vi "getGraph.vi"(0 "Cam_Calib_file":path, 1 "Spec_Calib_file":path, 3 "ROI":bool, 4 "map":path, 5 "y0":i32, 6 "FW":bool, 7 "image in":path, 9 "cam (0,1,2,3)":i32, 10 "Lens":string(combo)="f8x06", 11 "Image Name":string, 12 "B [T]":dbl=1.0) -> (13 "output cluster":cluster{"dp [MeV/C]":dbl[], dbl[]}(graph), 14 "Y":dbl[][](array[numeric]), 15 "X":dbl[][](array[numeric]), 17 "Momentum [MeV/C]":dbl[](graph), 18 "z":dbl[][](array[numeric]), 19 "pixel angel (y)":dbl[](graph)=[0.28800769934064135, 0.2882095085032147, 0.2884115340157437, 0.28861377619454537, 0.2888162353565284, 0.2890189118191943, 0.2892218059006397, 0.289423234715329, 0.2896096026494926, 0.2897858413876203, 0.28996224180170876, 0.29013880409125165, 0.2903155284560538, 0.2904924150962318, 0.29066946421221485, 0.2908466760047451, 0.2910240506748785, 0.2912200888475889, 0.29142082546369963, 0.29162177442700027, 0.2918229360446737, 0.29202431062447265, 0.2922258984747208, 0.29242769990431444, 0.2926297152227232, 0.29283191570579953, 0.2930334377606523, 0.2932351725330019, 0.2934371203297612, 0.2936387877464904, 0.2938402641743795, 0.2940419529321517, 0.2942438543260385, 0.29444596866283795, 0.2946480589358109, 0.29484968035757747, 0.29505151355782316, 0.2952535588408159, 0.2954558165113846, 0.29565828687491924, 0.2958609702373737, 0.2960638669052662, 0.2962669771856805, 0.2964698040291343, 0.2966723158133113, 0.2968750398090262, 0.2970779763202955, 0.2972811256516943, 0.29748448810835737, 0.29768806399598025, 0.29789287923215024, 0.29809853177062107, 0.2982861778747611, 0.2984666288230578, 0.2986472437516359, 0.29882802286022364, 0.2990089663488561, 0.2991900744178752, 0.29937134726793113, 0.2995527850999821, 0.29973438811529546, 0.2999384554163026, 0.3001441852119658, 0.30035013071239275, 0.30055629222582286, 0.300762670061059, 0.3009692645274684, 0.3011760759349845, 0.3013831045941078, 0.30159015680064977, 0.30179572710684616, 0.3019980055244977, 0.3022004922691996, 0.30240318763470797, 0.30260609191531024, 0.3028092054058265, 0.30301252840161114, 0.30321606119855377, 0.3034193370385415, 0.303622099252708, 0.3038250695143296, 0.30402824811549045, 0.30423163534880104, 0.30443523150739876, 0.3046390368849498, 0.3048430517756495, 0.30504727647422436, 0.305250926214299, 0.30545430210508306, 0.30565724830341984, 0.3058593076106099, 0.3060615723804524, 0.3062640428992535, 0.3064667194538319, 0.30666960233151963, 0.3068726918201636, 0.3070747819785802, 0.3072768576621269, 0.30747913769575613, 0.30768162236242985, 0.30788431194561355, 0.30808720672927653, 0.3082903069978933, 0.3084936130364445, 0.3086970146579123, 0.30889922498337297, 0.3091016386512774, 0.30930519276357565, 0.30950964116951185, 0.30971429656540866, 0.30991915923741287, 0.31012422947217805, 0.31032950755686545, 0.31052667203082357, 0.3107046103456832, 0.31088270164873605, 0.31106094611610596, 0.31123934392417213, 0.31141789524956964, 0.3115966002691897, 0.31177545916018046, 0.3119544720999468, 0.31214640622298384, 0.31234998693136795, 0.31255336482074314, 0.31275519333119467, 0.31295722155025546, 0.31315944974786275, 0.3133618781944213, 0.31356450716080464, 0.3137673369183555, 0.3139684633147784, 0.3141691648118955, 0.31437006254733935, 0.31457115678279784, 0.31477244778040603, 0.3149739358027459, 0.3151756211128486, 0.31537750397419384, 0.3155795846507125, 0.3157784918983376, 0.3159787797187646, 0.31617965487765226, 0.31638072445801957, 0.31658198871544435, 0.31678344790593305, 0.3169851022859213, 0.3171869521122753, 0.317387977202208, 0.3175852989941981, 0.31778280689627375, 0.3179805011460661, 0.3181783819815921, 0.31837644964125583, 0.31857470436384855, 0.3187731463885496, 0.31897177595492787, 0.319164425005991, 0.3193518219719201, 0.3195393858305189, 0.3197271167829648, 0.319915015030744, 0.32010308077565147, 0.32029131421979173, 0.32047971556557964, 0.3206682850157408, 0.3208688467868947, 0.3210756600957864, 0.3212826784341325, 0.3214899020805093, 0.3216973313139795, 0.3219049664140931, 0.3221128076608881, 0.32232085533489246, 0.322529109717124, 0.3227113886977328, 0.3228905273030448, 0.3230698154730057, 0.3232492533752553, 0.3234288411776704, 0.3236085790483658, 0.3237884671556941, 0.3239685056682464, 0.3241511143038239, 0.3243524891978669, 0.3245540552936161, 0.3247552106478079, 0.3249552231079993, 0.32515542436888734, 0.32535581467399116, 0.32555639426723304, 0.32575716339293825, 0.32596597642227865, 0.3261901232146414, 0.3264145104321994, 0.3266391384324378, 0.32686400757353024, 0.3270891182143402, 0.327314470714423, 0.32754006543402703, 0.32776590273409556, 0.32799189932134853, 0.3282180755480182, 0.32844449509892426, 0.32867115833698873, 0.3288980656258346, 0.3291252173297875, 0.32935261381387765, 0.32958025544384106, 0.32980814258612173, 0.330028974231201, 0.33024815924312484, 0.33046756988987364, 0.3306872937363768, 0.3309074671757531, 0.33112786774508135, 0.33134849576745934, 0.3315693515665783, 0.331790255775179, 0.3320036146728935, 0.3322171849209621, 0.33243096680671685, 0.33264496061799237, 0.3328591666431264, 0.33307358517096125, 0.333288216490845, 0.3335030608926323, 0.3337238815649635, 0.33396228506727366, 0.3342009553991622, 0.3344398929760186, 0.3346790982140716, 0.3349185715303916, 0.335158313342892, 0.33539832407033227, 0.3356386041323192, 0.33586336923097243, 0.3360709979838858, 0.33627882311063856, 0.3364836936146091, 0.3366885950037914, 0.33689368820826937, 0.3370989734740675, 0.33730445104761525, 0.33751012117574847, 0.3377137462769637, 0.3379166145664905, 0.33811966975822294, 0.3383229120876115, 0.3385263417904872, 0.3387299591030621, 0.33893376426193, 0.3391377575040679, 0.3393419390668357, 0.33957117083159105, 0.3398025156289204, 0.3400341070851385, 0.3402659455657455, 0.3404980314369444, 0.3407303650656422, 0.34096294681945183, 0.3411957770666942, 0.34142339852169173, 0.3416239795756783, 0.341824740848181, 0.3420256825600719, 0.34222680493256974, 0.34242810818724057, 0.34262959254599806, 0.3428312582311045, 0.3430331054651715, 0.34323429066279754, 0.3434343003072502, 0.3436344879226952, 0.3438348537248517, 0.3440353979297727, 0.3442361207538469, 0.3444370224137983, 0.3446381031266871, 0.34483936310991076, 0.3450578626541485, 0.3452874643561488, 0.3455173043193103, 0.34574732020818016, 0.3459723897434692, 0.3461976898022912, 0.34642322071410303, 0.346648982808974, 0.34687497641758697, 0.34707394456279084, 0.34726779758963844, 0.3474618167179976, 0.3476560021425361, 0.34785035405821507, 0.34804487266028833, 0.34823955814430335, 0.3484344107061026, 0.3486312649180983, 0.34885495465101213, 0.3490788695629513, 0.3493030099695635, 0.34952737618707086, 0.3497519685322719, 0.34997731548961586, 0.35020527925995326, 0.35043347490544124, 0.35065231866296387, 0.3508480345697342, 0.3510439168590296, 0.3512399657230985, 0.3514361813544731, 0.3516325639459694, 0.3518291136906883, 0.3520258307820155, 0.3522227154136226, 0.35241870033027983, 0.35261385771009734, 0.3528091794518836, 0.35300466574353223, 0.3532003167732107, 0.3533961327293609, 0.35359211380069955, 0.35378793248579343, 0.3539823127088366, 0.35419856946847766, 0.3544224703728747, 0.3546465920460918, 0.3548709347899404, 0.3550954989067666, 0.35532028469945204, 0.355545292471415, 0.3557705225266119, 0.35599597516953835, 0.3562195465688293, 0.35644327578022983, 0.3566672238740321, 0.35689139114683444, 0.35711577789575555, 0.35734038441843524, 0.357565211013036, 0.3577868369248013, 0.3579969740834651, 0.3581801509931798, 0.3583634719989251, 0.35854693725604614, 0.3587305469201026, 0.35891430114686995, 0.35909820009233984, 0.35928224391272, 0.35946643276443463, 0.35966343275620455, 0.3598777096374909, 0.36009218772835716, 0.3603068672927925, 0.3605217485952368, 0.3607368319005817, 0.36095458016808163, 0.36117878865288006, 0.3614032134202907, 0.36160546206413874, 0.36179594817013894, 0.3619865861077824, 0.36217737604056577, 0.36236831813220927, 0.362559412546657, 0.36275065944807766, 0.3629420590008647, 0.36313361136963646, 0.363351808428183, 0.3635738459612016, 0.36379609356232473, 0.3640185515055202, 0.36423767597445017, 0.364450336432046, 0.36466319251442797, 0.36487624447297334, 0.36508925281984417, 0.36530043816401897, 0.365511815657225, 0.36572338554338923, 0.36593514806684124, 0.3661471034723142, 0.3663592520049456, 0.3665715939102782, 0.3667841294342608, 0.3669960968480711, 0.367206729858304, 0.3674198832826266, 0.3676334264586519, 0.36784716366746734, 0.3680610951539646, 0.3682752211634362, 0.3684895419415763, 0.36870405773448195, 0.36889898923916287, 0.36907852436519195, 0.3692581922210982, 0.3694379929399495, 0.36961792665498383, 0.36979799349960923, 0.36997791071534186, 0.37015298423759135, 0.37032818465487666, 0.370527824153792, 0.370734224899929, 0.37094080653068184, 0.37114756926726766, 0.3713545133312559, 0.3715616389445682, 0.3717689463294794, 0.3719764357086188, 0.3721840747166905, 0.3723895491590272, 0.3725955361453253, 0.37280376147382954, 0.3730121687603038, 0.37322075822564516, 0.3734295300910985, 0.3736384845782571, 0.37384762190906357, 0.37405635571757884, 0.3742634182839463, 0.37447065975982285, 0.37467808035967864, 0.37488568029831626, 0.3750934597908729, 0.3753031816848105, 0.37551380655424726, 0.37572461515960376, 0.3759344528378446, 0.37614315553648375, 0.37635203799113537, 0.3765611004155991, 0.3767703430240029, 0.3769797660308043, 0.37718936965079053, 0.37739915409907876, 0.3776091195911178, 0.3778123048177794, 0.3780130727617814, 0.3782140080126384, 0.37841511076446727, 0.3786163812116777, 0.3788178195489723, 0.3790194259713473, 0.37922120067409315, 0.37942314385279496, 0.37959132786416794, 0.3797567204840217, 0.37992360723587615, 0.3800914896866685, 0.38025948438880225, 0.3804275914436931, 0.3805958109528732, 0.380764143017991, 0.38093731804963116, 0.3811378564602311, 0.38133855908668424, 0.3815394261150738, 0.3817404577317556, 0.38194370958430596, 0.38214741221894494, 0.3823512831791136, 0.3825553226566906, 0.3827585341269448, 0.38296024944966484, 0.3831621291366564, 0.3833641733723683, 0.3835663823415161, 0.38376875622908285, 0.3839664488014421, 0.38415997372343197, 0.38435365206763583, 0.3845668564899877, 0.38479308272283114, 0.38501952376050674, 0.3852461798925063, 0.3854730514088339, 0.3857001386000069, 0.3859274417570573, 0.3861568553104828, 0.3863866526183244, 0.3865851388515057, 0.3867772598985196, 0.3869695298488373, 0.3871619488624852, 0.3873545170997119, 0.3875472347209896, 0.38774010188701397, 0.38793081685388153, 0.38812024927651523, 0.3883072180685801, 0.3884943280128661, 0.3886815792576781, 0.38886897195152265, 0.38905650624310933, 0.3892441822813508, 0.38943200021536284, 0.3896199601944651, 0.3898072824309816, 0.3899927621065785, 0.39017837977852254, 0.39036413558945854, 0.39055002968222213, 0.39073606219984064, 0.39092223328553327, 0.39110717852291554, 0.39129003029545684, 0.3914716422770283, 0.39165206132783087, 0.39183261109100753, 0.3920132916986519])   [LabVIEW 2011]
uses:
  <vilib>/vision/NI_Vision_Development_Module.lvlib
panel:
  out "Image Pixels (I16)":i16[][](graph)
  out "start":dbl
  in  "Cluster":cluster{"0":i32, "1":i32, "2":i32, "3":i32}
  out "x/y":dbl[][](graph)
  out "filenames":string[](array[string])
  out "Image Dst Out":T1(plugin-control)
  out "Y Resolution":i32
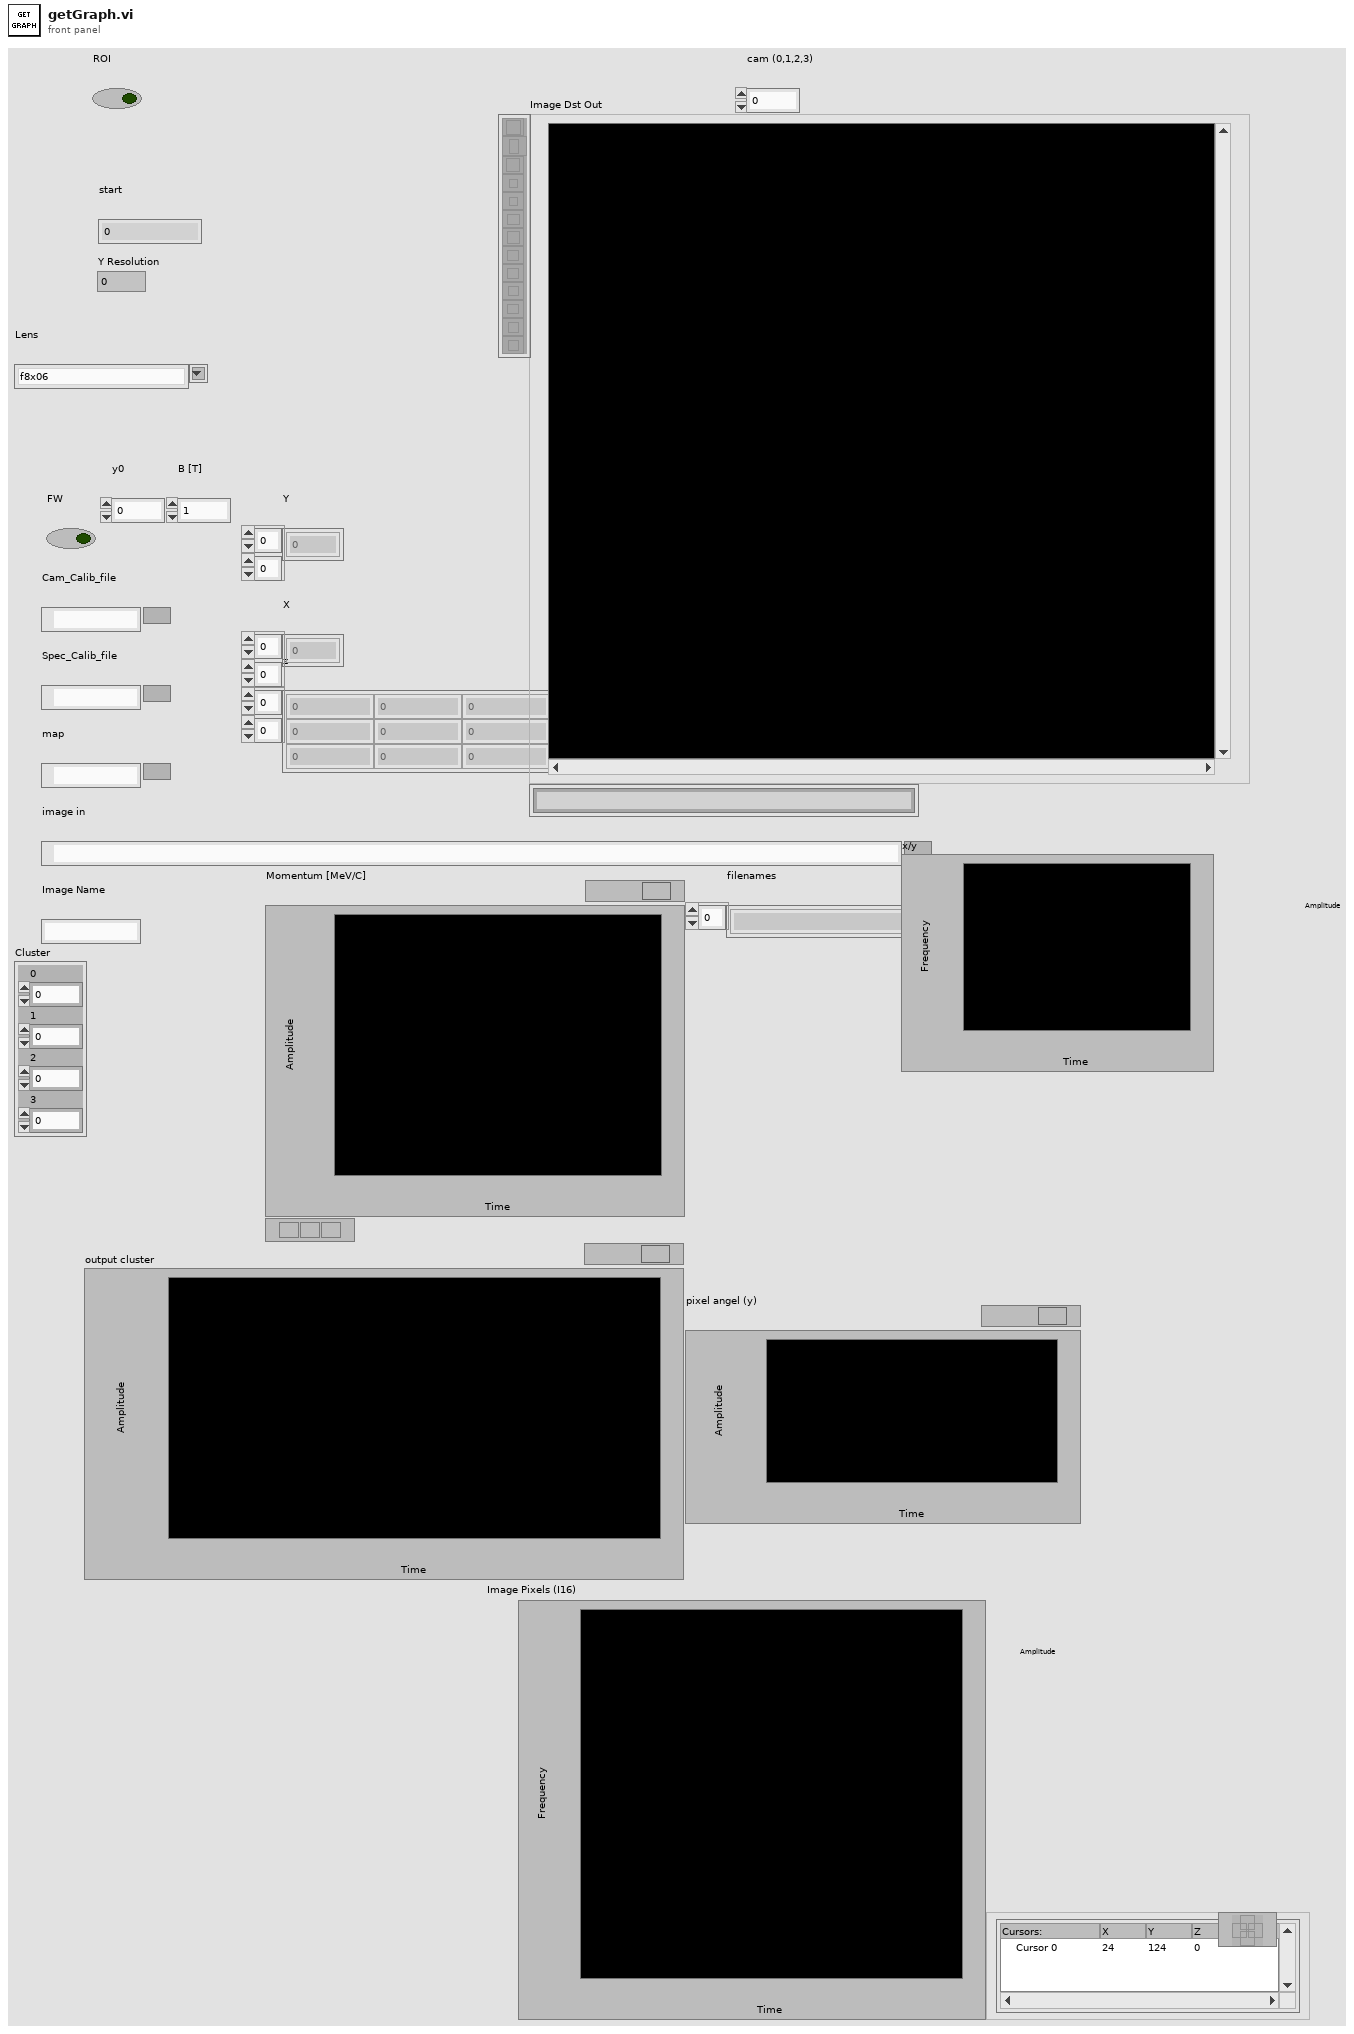
[diagram p1: front panel]
types:
  T1 = typedef "IMAQ Image.ctl" = refnum<image>
  T2 = cluster{"X Size":i32, "Y Size":i32, "Order #":i32}
  T3 = cluster{"npix-X":i32, "npix-Y":i32, "Left [pix]":dbl, "Top [pix]":dbl}
  T4 = cluster{"Screen Orientation":string, "Screen angle":string, "Lens":string, "Calibration (mm/pix)":dbl}
  T5 = typedef "Image Type" = u32
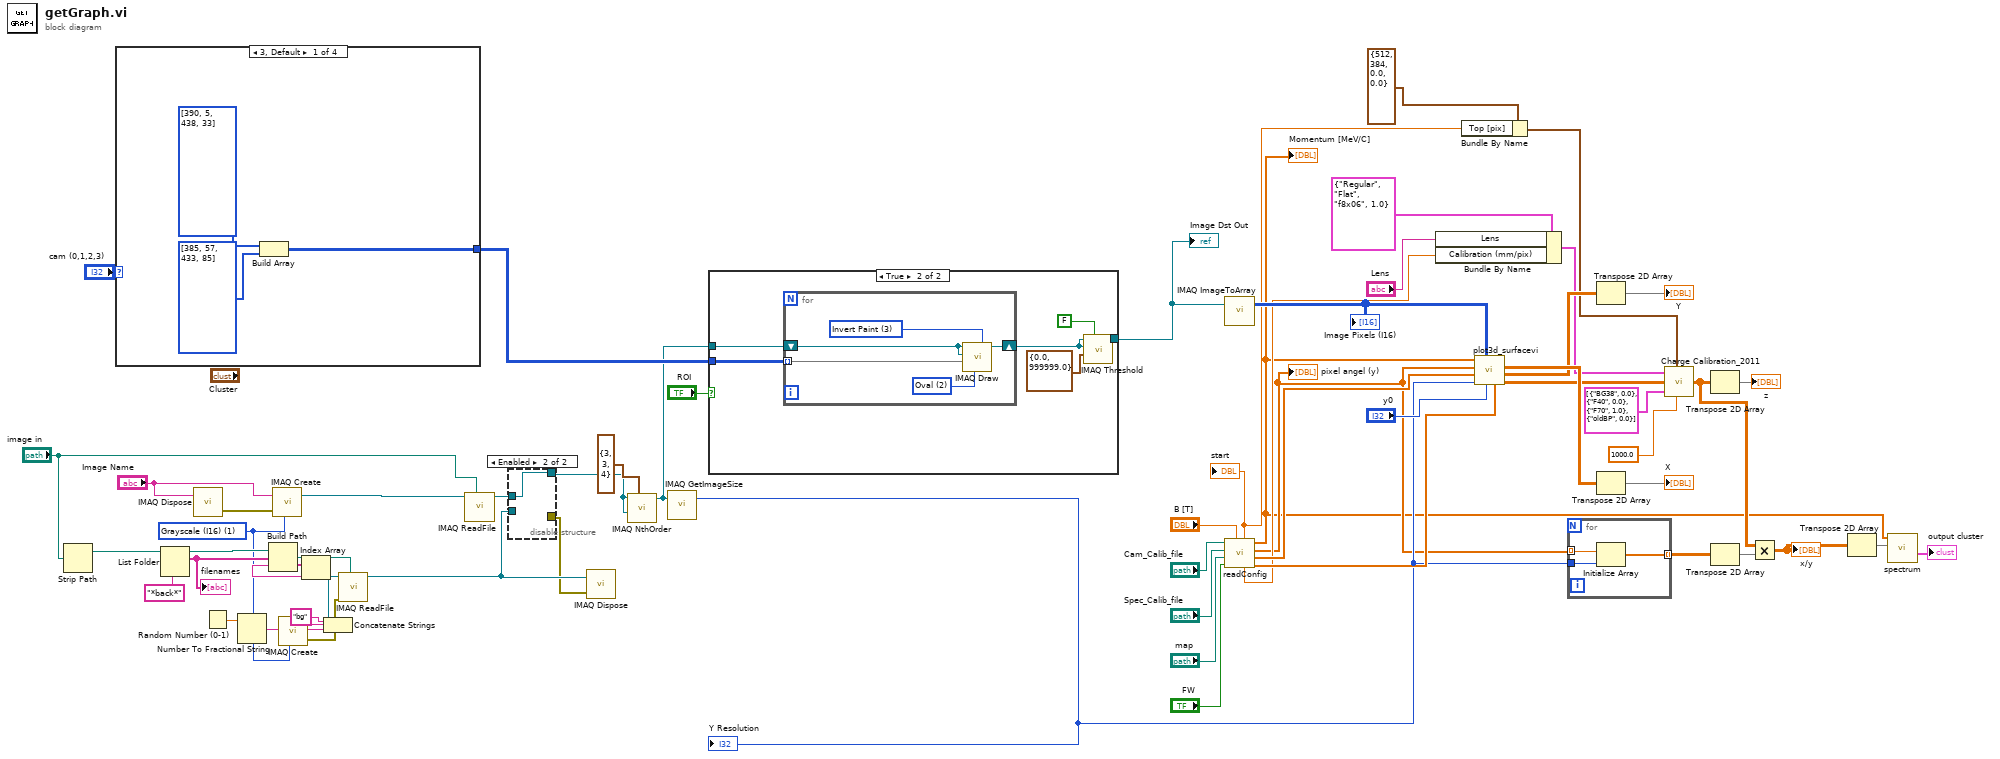
[diagram p0: block diagram]
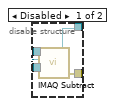
[diagram p2: hidden frame]
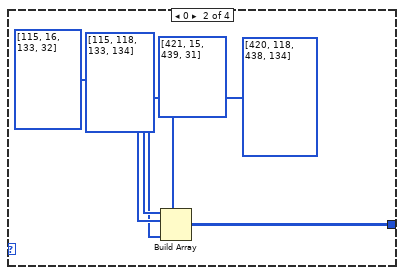
[diagram p3: hidden frame]
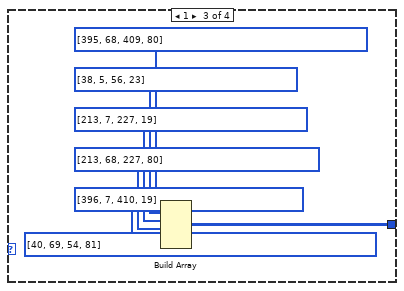
[diagram p4: hidden frame]
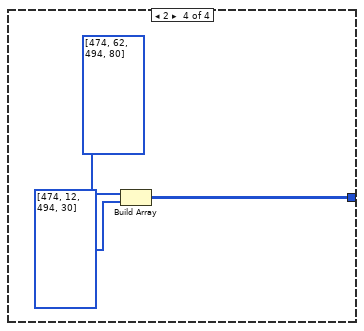
[diagram p5: hidden frame]
diagram:
  w22 = T5 1 items=["Grayscale (U8)", "Grayscale (I16)", "Grayscale (SGL)", "Complex (CSG)", "RGB (U32)", "HSL (U32)", "RGB (U64)", "Grayscale (U16)"] ("Image Type")
  n1 = Strip Path(path="image in") -> (stripped path=w31:path)  [unwired: 1 out]
  n2 = case shown="3, Default" "cam (0,1,2,3)" {
    tunnel: [w61 w66 w73 w76] -> w13
    frame 3, Default {
      n3 = Build Array(i32[] [390, 5, 438, 33] ("Points"), i32[] [385, 57, 433, 85] ("Points")) -> (w61:i32[][])
    }
    frame 0 {
      n4 = Build Array(i32[] [115, 16, 133, 32] ("Global Rectangle"), i32[] [115, 118, 133, 134] ("Global Rectangle"), i32[] [421, 15, 439, 31] ("Global Rectangle"), i32[] [420, 118, 438, 134] ("Global Rectangle")) -> (w66:i32[][])
    }
    frame 1 {
      n5 = Build Array(i32[] [395, 68, 409, 80] ("Global Rectangle"), i32[] [38, 5, 56, 23] ("Global Rectangle"), i32[] [213, 7, 227, 19] ("Global Rectangle"), i32[] [213, 68, 227, 80] ("Global Rectangle"), i32[] [396, 7, 410, 19] ("Global Rectangle"), i32[] [40, 69, 54, 81] ("Global Rectangle")) -> (w73:i32[][])
    }
    frame 2 {
      n6 = Build Array(i32[] [474, 62, 494, 80] ("Points"), i32[] [474, 12, 494, 30] ("Points")) -> (w76:i32[][])
    }
  }
  n7 = List Folder(path=w31, pattern="*back*") -> (path out=w28:path, filenames=w29:string[])  [unwired: 2 in, 2 out]
  "filenames" <- w29
  n8 = call "IMAQ Dispose"("Image"="Image Name") -> ("error out"=w54:errorcluster)  [unwired: 5 in]
  n9 = Random Number (0-1)() -> (number: 0 to 1=w26:dbl)
  n10 = Number To Fractional String(number=w26) -> (F-format string=w24:string)  [unwired: 3 in]
  n11 = call "IMAQ Create"("Image Name"="Image Name", "Image Type"=w22, "error in (no error)"=w54) -> ("New Image"=w52:T1)  [unwired: 2 in, 1 out]
  n12 = Index Array(array=w29) -> (element=w27:string)  [unwired: 1 in]
  n13 = Build Path(base path=w28, name or relative path=w27) -> (appended path=w20:path)
  n14 = Concatenate Strings("bg" ("Image Name"), w24) -> (w23:string)
  n15 = call "IMAQ Create"("Image Name"=w23, "Image Type"=w22) -> ("New Image"=w21:T1, "error out"=w17:errorcluster)  [unwired: 3 in]
  n16 = call "IMAQ ReadFile"("File Path"=w20, "error in (no error)"=w17, "Image"=w21) -> ("Image Out"=w16:T1)  [unwired: 4 in, 4 out]
  n17 = call "IMAQ ReadFile"("File Path"="image in", "Image"=w52) -> ("Image Out"=w19:T1)  [unwired: 5 in, 4 out]
  n18 = disable-structure shown="Enabled" {
    disable-tunnel: w19 -> [w82 w83]
    disable-tunnel: [w81 w83] -> w18
    disable-tunnel: w16 -> [w80 _]
    disable-tunnel: [w79 _] -> w15
    frame Disabled {
      n19 = call "IMAQ Subtract"("Image Src A"=w82, "Image Dst"=w82, "Image Src B"=w80) -> ("Image Dst Out"=w81:T1, "error out"=w79:errorcluster)  [unwired: 4 in]
    }
    frame Enabled {
    }
  }
  n20 = call "IMAQ Dispose"("Image"=w16, "error in (no error)"=w15) -> ()  [unwired: 4 in, 1 out]
  n21 = call "IMAQ NthOrder"("Image Src"=w18, "Size & Order #"=T2 {"X Size"=3, "Y Size"=3, "Order #"=4}, "Image Dst"=w18) -> ("Image Dst Out"=w1:T1)  [unwired: 4 in, 1 out]
  n22 = call "IMAQ GetImageSize"("Image"=w1) -> ("Y Resolution"=w12:i32)  [unwired: 3 in, 2 out]
  "Y Resolution" <- w12
  n23 = case shown="True" "ROI" {
    tunnel: w1 -> [w84 w88]
    tunnel: [w84 w87] -> w2
    tunnel: w13 -> [_ w85]
    frame False {
    }
    frame True {
      n24 = for {
        shift-right: [w94] -> w86
        shift-left: w88 -> [w95]
        tunnel: w85 -> [w91] mode=indexing
        w93 = u16 2 items=["Line", "Rectangle", "Oval"] ("Shape to draw")
        w92 = u16 3 items=["Frame", "Paint", "Invert Frame", "Invert Paint"] ("Draw Mode")
        n25 = call "IMAQ Draw"("Draw Mode"=w92, "Shape to draw"=w93, "Coordinates"=w91, "Image Dst"=w95, "Image Src"=w95) -> ("Image Dst Out"=w94:T1)  [unwired: 5 in, 1 out]
      }
      n26 = call "IMAQ Threshold"("Keep/Replace Value (Replace)"=FALSE, "Range"=cluster{"Lower value":sgl, "Upper value":sgl} {"Lower value"=0.0, "Upper value"=999999.0}, "Image Dst"=w86, "Image Src"=w86) -> ("Image Dst Out"=w87:T1)  [unwired: 6 in, 1 out]
    }
  }
  "Image Dst Out" <- w2
  n27 = call "IMAQ ImageToArray"("Image"=w2) -> ("Image Pixels (I16)"=w55:i16[][])  [unwired: 3 in, 4 out]
  "Image Pixels (I16)" <- w55
  n28 = call "readConfig.vi"("B [T]"="B [T]", "FW"="FW", "map"="map", "Spec_Calib_file"="Spec_Calib_file", "Cam_Calib_file"="Cam_Calib_file") -> ("charge compensation"=w50:dbl[], "dp [MeV/C]"=w60:dbl[], "pixel angel (y)"=w11:dbl[], "Momentum [MeV/C]"=w6:dbl[], "field of view /pixel"=w41:dbl, "start"=w37:dbl)  [unwired: 1 in]
  "pixel angel (y)" <- w11
  "Momentum [MeV/C]" <- w6
  "start" <- w37
  n29 = Bundle By Name(cluster=T4 {"Screen Orientation"="Regular", "Screen angle"="Flat", "Lens"="f8x06", "Calibration (mm/pix)"=1.0} ("Screen&Camera 2"), "Lens"="Lens", "Calibration (mm/pix)"=w41) -> (w40:T4)
  n30 = Bundle By Name(cluster=T3 {"npix-X"=512, "npix-Y"=384, "Left [pix]"=0.0, "Top [pix]"=0.0} ("ROI infos"), "Top [pix]"=w37) -> (w36:T3)
  n31 = call "plot3d_surfacevi.vi"("charge compensation"=w50, "y0"="y0", "Image Pixels (I16)"=w55, "y size"=w12, "dp [MeV/C]"=w60, "pixel angel (y)"=w11, "Momentum [MeV/C]"=w6) -> ("z"=w14:dbl[][], "Y"=w46:dbl[][], "X"=w48:dbl[][])  [unwired: 2 in]
  n32 = for {
    tunnel: w11 -> [w98] mode=indexing
    tunnel: [w97] -> w8 mode=indexing
    tunnel: w12 -> [w96]
    n33 = Initialize Array(w98, w96) -> (w97:dbl[])
  }
  n34 = Transpose 2D Array(2D array=w46) -> (transposed array=→"Y":dbl[][])
  n35 = Transpose 2D Array(2D array=w48) -> (transposed array=→"X":dbl[][])
  n36 = call "Charge Calibration_2011.vi"("Screen&Camera"=w40, "ROI infos"=w36, "Image (Counts)"=w14, "Filters"=cluster{"Name":string, "#Filters":dbl}[] [{"Name"="BG38", "#Filters"=0.0}, {"Name"="F40", "#Filters"=0.0}, {"Name"="F70", "#Filters"=1.0}, {"Name"="oldBP", "#Filters"=0.0}], "Electron energy (MeV)"=1000.0) -> ("Image (pC)"=w9:dbl[][])  [unwired: 4 in]
  n37 = Transpose 2D Array(2D array=w9) -> (transposed array=→"z":dbl[][])
  n38 = Transpose 2D Array(2D array=w8) -> (transposed array=w7:dbl[][])
  n39 = Multiply(x=w9, y=w7) -> (x*y=w4:dbl[][])
  "x/y" <- w4
  n40 = Transpose 2D Array(2D array=w4) -> (transposed array=w3:dbl[][])
  n41 = call "spectrum.vi"("z in"=w3, "Momentum [MeV/C]"=w6) -> ("output cluster"=→"output cluster":cluster{"dp [MeV/C]":dbl[], dbl[]})  [unwired: 9 in]
